vi "5.4.vi"() -> ()   [LabVIEW 2023]
uses:
  <vilib>/addons/control/pid/NI_PID_pid.lvlib
  <vilib>/addons/control/pid/pid.llb/PID Gain Schedule (DBL).vi
  <vilib>/addons/control/pid/pid.llb/PID (DBL).vi
panel:
  out "Waveform Chart":dbl(graph)
  in  "stop":bool
  in  "PID gain schedule":T1(array[cluster])=[{"PID gains"={"proportional gain (Kc)"=1.0, "integral time (Ti, min)"=0.01, "derivative time (Td, min)"=0.0}, "max value"=100.0}] {"max value" format="%.2f"; "PID gains"."derivative time (Td, min)" format="%.3f"; "PID gains"."integral time (Ti, min)" format="%.3f"; "PID gains"."proportional gain (Kc)" format="%.3f"}
  out "PID Output":dbl
  out "Duty Cycle":dbl
  in  "Setpoint":dbl
  out "m/s":dbl
  out "Vong/s":dbl
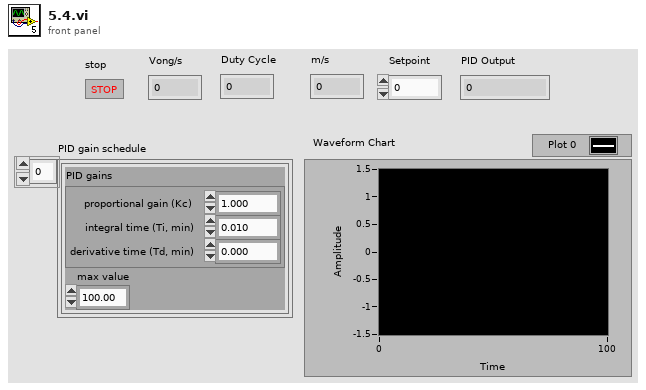
[diagram p1: front panel]
types:
  T1 = cluster{"PID gains":cluster{"proportional gain (Kc)":dbl, "integral time (Ti, min)":dbl, "derivative time (Td, min)":dbl}, "max value":dbl}[]
  T2 = cluster{"proportional gain (Kc)":dbl, "integral time (Ti, min)":dbl, "derivative time (Td, min)":dbl}
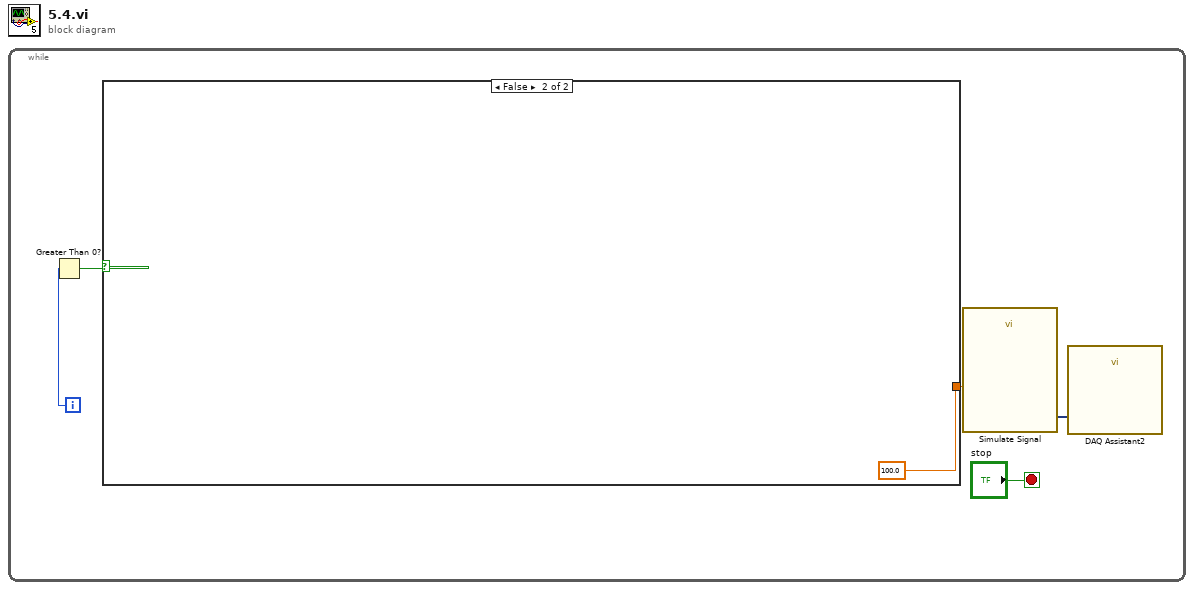
[diagram p0: block diagram]
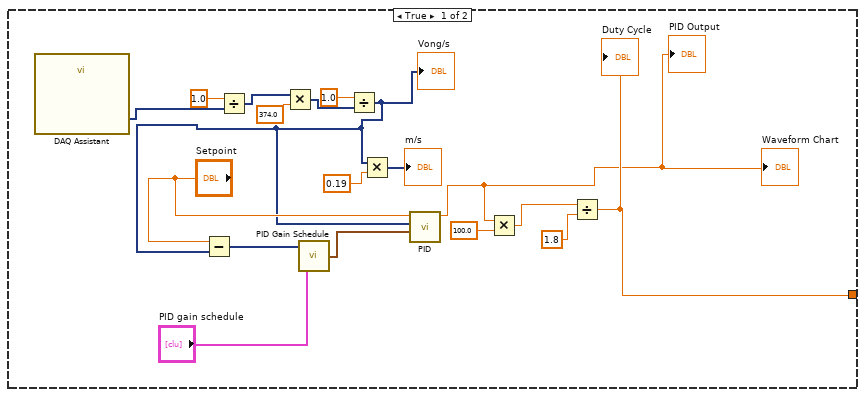
[diagram p2: hidden frame]
diagram:
  n1 = while {
    i -> [w3]
    stop <- "stop" stop-if-true
    n2 = Greater Than 0?(x=w3) -> (x > 0?=w2:bool)
    n3 = case shown="False" w2 {
      tunnel: [w8 100.0] -> w5
      frame True {
        n4 = call "DAQ Assistant"() -> ("data"=w23:dynamicdata)  [unwired: 17 in, 2 out]
        n5 = Divide(x=1.0, y=w23) -> (x/y=w21:dynamicdata)
        n6 = Multiply(x=w21, y=374.0) -> (x*y=w19:dynamicdata)
        n7 = Divide(x=1.0, y=w19) -> (x/y=w12:dynamicdata)
        "Vong/s" <- w12
        n8 = Subtract(x="Setpoint", y=w12) -> (x-y=w15:dynamicdata)
        n9 = call-poly <vilib>:"PID Gain Schedule.vi"("PID gain schedule"="PID gain schedule", "gain scheduling value"=w15) -> ("PID gains out"=w13:T2)  [unwired: 2 in, 1 out]
        n10 = Multiply(x=w12, y=0.19) -> (x*y=→"m/s":dynamicdata)
        n11 = call-poly <vilib>:"PID.vi"("PID gains"=w13, "process variable"=w12, "setpoint"="Setpoint") -> ("output"=w6:dbl)  [unwired: 7 in, 1 out]
        "PID Output" <- w6
        "Waveform Chart" <- w6
        n12 = Multiply(x=w6, y=100.0) -> (x*y=w10:dbl)
        n13 = Divide(x=w10, y=1.8) -> (x/y=w8:dbl)
        "Duty Cycle" <- w8
      }
      frame False {
      }
    }
    n14 = call "Simulate Signal"("Duty Cycle (%)"=w5) -> ("Square with Uniform Noise"=w4:dynamicdata)  [unwired: 13 in, 1 out]
    n15 = call "DAQ Assistant2"("data"=w4) -> ()  [unwired: 16 in, 3 out]
  }
